vi "SwerveChooseCenter.vi"(6 "Defensive Driving Trigger":bool, 8 "Joystick Y":dbl, 9 "Joystick X":dbl) -> (3 "Center Choice":T1(ring))   [LabVIEW 2019]
doc: "This VI chooses a corner of the robot to pivot about during evasive manuervers based on the driver's current joystick commands."
uses:
  9a94878a-4914-4fba-839a-7657b048eec0.vi
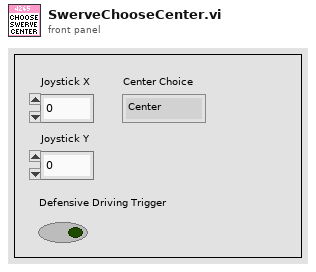
[diagram p1: front panel]
types:
  T1 = enum16{"Center", "Module 0", "Module 1", "Module 2", "Module 3"}
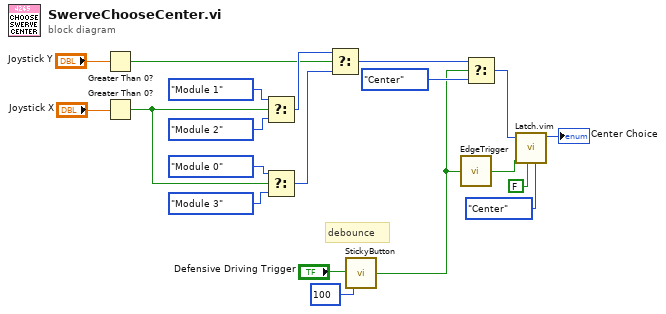
[diagram p0: block diagram]
diagram:
  # "debounce"
  n1 = Greater Than 0?(x="Joystick Y") -> (x > 0?=w17:bool)
  n2 = Greater Than 0?(x="Joystick X") -> (x > 0?=w19:bool)
  n3 = Select(t=T1."Module 1", s=w19, f=T1."Module 2") -> (s? t:f=w18:T1)
  n4 = Select(t=T1."Module 0", s=w19, f=T1."Module 3") -> (s? t:f=w20:T1)
  n5 = Select(t=w18, s=w17, f=w20) -> (s? t:f=w10:T1)
  n6 = call "StickyButton.vi"("Time threshold (ms)"=u32 100, "Button Input"="Defensive Driving Trigger") -> ("Sticky Button"=w1:bool)
  n7 = call "EdgeTrigger.vi"("Input Signal"=w1) -> ("All Edge Trigger"=w4:bool)  [unwired: 2 out]
  n8 = Select(t=w10, s=w1, f=T1."Center") -> (s? t:f=w12:T1)
  n9 = call "Latch.vim"("Default Value"=T1."Center", "Reset"=FALSE, "Latch Signal"=w4, "Latch Value"=w12) -> ("Latched"=→"Center Choice":T1)  [unwired: 7 in]
